vi "MSEncoder SubVI WriteWfm_PermanentCheck.vi"(4 "Access Permanent? (F)":bool, 5 "WfmData":dbl[](array[numeric]), 6 "AccessNewData? (F)":bool, 7 "xml string":string, 8 "error in (no error)":errorcluster, 9 "UpdIndex":i32, 11 "tdms file out":refnum<k34>) -> (0 "error out":errorcluster)   [LabVIEW 2018, in "MSEncoder.lvclass"]
uses:
  MSEncoder.lvclass
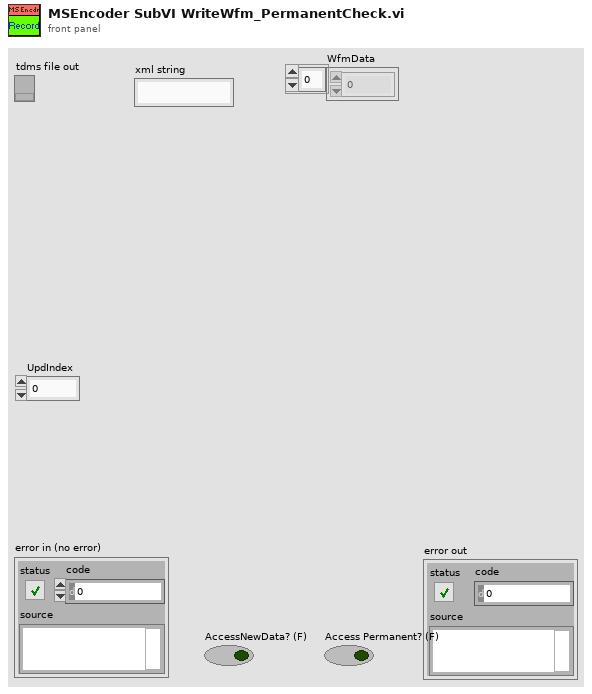
[diagram p1: front panel]
types:
  T1 = enum16{"open", "replace", "create", "open or create", "replace or create", "replace or create with confirmation"}
  T2 = enum16{"open", "open or create", "create or replace", "create", "open (read-only)"}
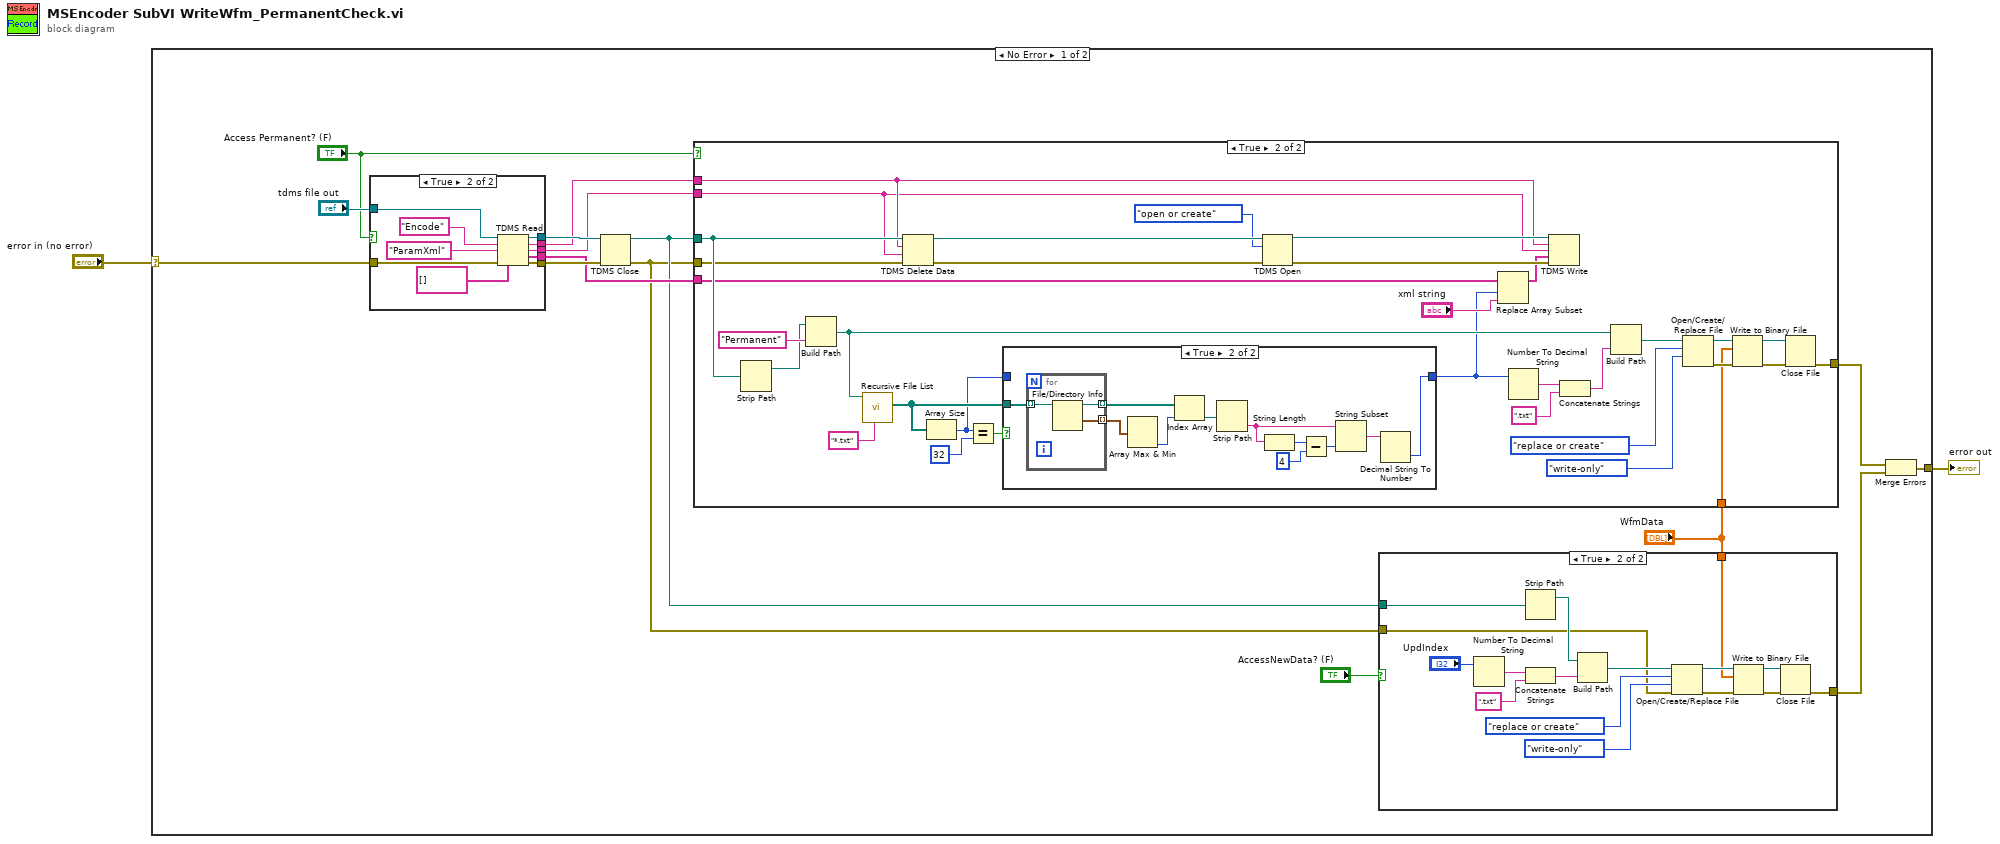
[diagram p0: block diagram]
diagram:
  n1 = case shown="No Error" "error in (no error)" {
    selector: "error in (no error)" -> [w3 w96]
    tunnel: [w6 w96] -> w2
    frame No Error {
      n2 = case shown="True" "Access Permanent? (F)" {
        tunnel: "tdms file out" -> [w18 w29]
        tunnel: [w18 w28] -> w15
        tunnel: [w19 w27] -> w14
        tunnel: [_ w26] -> w13
        tunnel: [_ w25] -> w12
        tunnel: [_ w23] -> w11
        tunnel: w3 -> [w19 w20]
        frame False {
        }
        frame True {
          n3 = TDMS Read(0:w29, 5:"Encode" ("group name in (Untitled)"), 7:"ParamXml" ("channel name(s) in (Untitled)"), 11:w20, 12:string[] []) -> (4:w28:refnum<k34>, 6:w26:string, 8:w25:string, 10:w23:string[], 15:w27:errorcluster)  [unwired: 3 in, 1 out]
        }
      }
      n4 = TDMS Close(8:w14, 11:w15) -> (0:w9:errorcluster, 3:w10:path)
      n5 = case shown="True" "Access Permanent? (F)" {
        tunnel: "WfmData" -> [_ w70]
        tunnel: w13 -> [_ w57]
        tunnel: w12 -> [_ w56]
        tunnel: w10 -> [_ w61]
        tunnel: w9 -> [w47 w60]
        tunnel: w11 -> [_ w55]
        tunnel: [w47 w48] -> w8
        frame False {
        }
        frame True {
          n6 = Strip Path(path=w61) -> (stripped path=w51:path)  [unwired: 1 out]
          n7 = Build Path(base path=w51, name or relative path="Permanent") -> (appended path=w50:path)
          n8 = call <vilib>:"Recursive File List.vi"("pattern"="*.txt", "Folder Path"=w50) -> ("All Files in Dir"=w69:path[])  [unwired: 5 in, 4 out]
          n9 = TDMS Delete Data(8:w60, 9:w56, 10:w57, 11:w61) -> (0:w62:errorcluster, 3:w64:path)  [unwired: 3 in]
          n10 = Array Size(array=w69) -> (size(s)=w68:i32)
          n11 = Equal?(x=w68, y=32) -> (x = y?=w67:bool)
          n12 = case shown="True" w67 {
            tunnel: w68 -> [w81 _]
            tunnel: [w81 w86] -> w49
            tunnel: w69 -> [_ w85]
            frame False {
            }
            frame True {
              n13 = for {
                tunnel: w85 -> [w95] mode=indexing
                tunnel: [w94] -> w84 mode=indexing
                tunnel: [w93] -> w83 mode=indexing
                n14 = File/Directory Info(path=w95) -> (path out=w93:path, last mod=w94:timestamp)  [unwired: 1 in, 5 out]
              }
              n15 = Array Max & Min(array=w84) -> (min index (indices)=w82:i32)  [unwired: 3 out]
              n16 = Index Array(array=w83, index=w82) -> (element=w92:path)
              n17 = Strip Path(path=w92) -> (name=w91:string)  [unwired: 1 out]
              n18 = String Length(string=w91) -> (length=w90:i32)
              n19 = Subtract(x=w90, y=4) -> (x-y=w88:i32)
              n20 = String Subset(string=w91, length (rest)=w88) -> (substring=w87:string)  [unwired: 1 in]
              n21 = Decimal String To Number(string=w87) -> (number=w86:i32)  [unwired: 2 in, 1 out]
            }
          }
          n22 = TDMS Open(8:w62, 10:T2."open or create" ("operation (0:open)"), 11:w64) -> (0:w58:errorcluster, 3:w59:refnum<k34>)  [unwired: 4 in]
          n23 = Replace Array Subset(array=w55, new element="xml string", index=w49) -> (w53:string[])
          n24 = Number To Decimal String(number=w49) -> (decimal integer string=w80:string)  [unwired: 1 in]
          n25 = TDMS Write(0:w59, 5:w57, 7:w56, 9:w53, 11:w58) -> ()  [unwired: 1 in, 4 out]
          n26 = Concatenate Strings(w80, ".txt" ("string")) -> (w78:string)
          n27 = Build Path(base path=w50, name or relative path=w78) -> (appended path=w77:path)
          n28 = Open/Create/Replace File(file path (use dialog)=w77, operation (0:open)=T1."replace or create", access (0:read/write)=enum16{"read/write", "read-only", "write-only"}."write-only") -> (refnum out=w74:refnum<file>, error out=w73:errorcluster)  [unwired: 3 in, 1 out]
          n29 = Write to Binary File(file (use dialog)=w74, data=w70, error in=w73) -> (refnum out=w72:refnum<file>, error out=w71:errorcluster)  [unwired: 3 in, 1 out]
          n30 = Close File(refnum=w72, error in=w71) -> (error out=w48:errorcluster)  [unwired: 1 out]
        }
      }
      n31 = case shown="True" "AccessNewData? (F)" {
        tunnel: "WfmData" -> [_ w35]
        tunnel: w10 -> [_ w33]
        tunnel: w9 -> [w30 w32]
        tunnel: [w30 w31] -> w7
        frame False {
        }
        frame True {
          n32 = Number To Decimal String(number="UpdIndex") -> (decimal integer string=w46:string)  [unwired: 1 in]
          n33 = Strip Path(path=w33) -> (stripped path=w34:path)  [unwired: 1 out]
          n34 = Concatenate Strings(w46, ".txt" ("string")) -> (w44:string)
          n35 = Build Path(base path=w34, name or relative path=w44) -> (appended path=w43:path)
          n36 = Open/Create/Replace File(file path (use dialog)=w43, error in=w32, operation (0:open)=T1."replace or create", access (0:read/write)=enum16{"read/write", "read-only", "write-only"}."write-only") -> (refnum out=w40:refnum<file>, error out=w39:errorcluster)  [unwired: 2 in, 1 out]
          n37 = Write to Binary File(file (use dialog)=w40, data=w35, error in=w39) -> (refnum out=w38:refnum<file>, error out=w37:errorcluster)  [unwired: 3 in, 1 out]
          n38 = Close File(refnum=w38, error in=w37) -> (error out=w31:errorcluster)  [unwired: 1 out]
        }
      }
      n39 = Merge Errors(w8, w7) -> (w6:errorcluster)
    }
    frame Error {
    }
  }
  "error out" <- w2
